vi "task.vi"() -> ()   [LabVIEW 2019]
uses:
  <vilib>/DAQmx/read.llb/DAQmx Read.vi
  <vilib>/DAQmx/read.llb/DAQmx Read (Analog 1D Wfm NChan NSamp).vi
  <vilib>/DAQmx/miscellaneous.llb/DAQmx Fill In Error Info.vi
panel:
  out "data":waveform(dbl)[](graph) caption="数据"
  in  "stop":bool caption="停止"
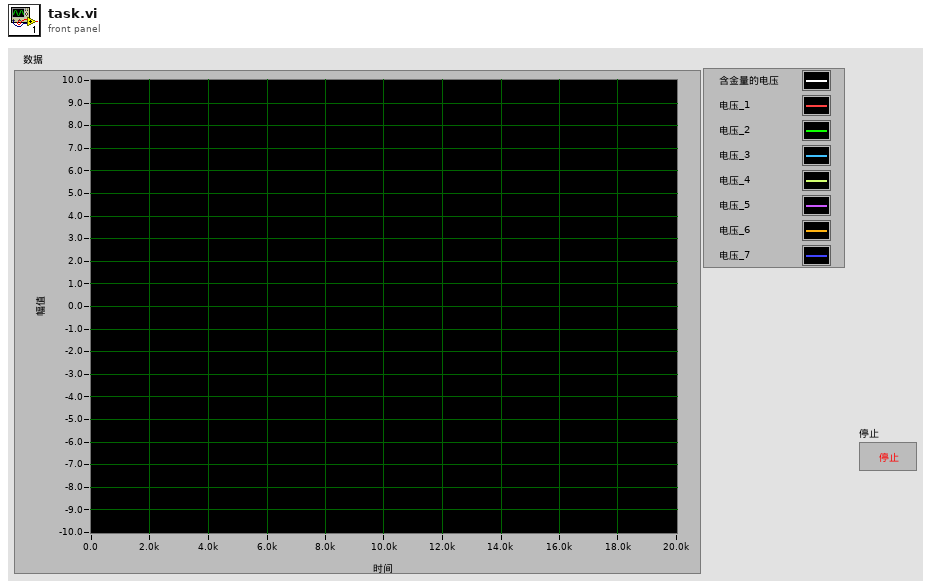
[diagram p1: front panel]
types:
  T1 = enum16{"open", "open or create", "create or replace", "create", "open (read-only)"}
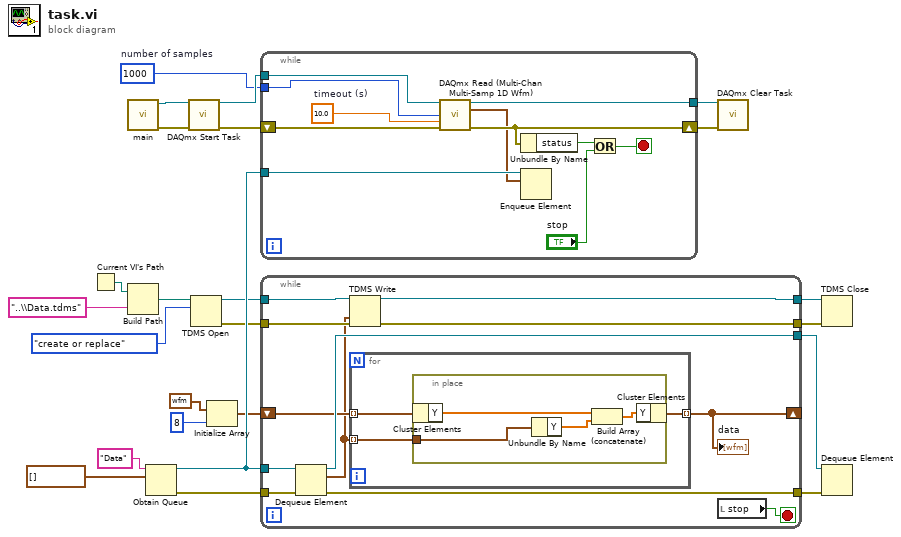
[diagram p0: block diagram]
diagram:
  w22 = 1000  # number of samples
  n1 = Current VI's Path() -> (path=w7:path)
  n2 = call "main.vi"() -> ("error out"=w18:errorcluster, "task out"=w19:refnum<k21>)  [unwired: 10 in]
  n3 = Build Path(base path=w7, name or relative path="..\\Data.tdms" ("名称或相对路径")) -> (appended path=w5:path)
  n4 = Obtain Queue(name (unnamed)="Data" ("名称（未命名）"), element data type=waveform(dbl)[] [] ("data")) -> (queue out=w14:refnum<queue>, error out=w15:errorcluster)  [unwired: 3 in, 1 out]
  n5 = call <vilib>:"DAQmx Start Task.vi"("task/channels in"=w19, "error in"=w18) -> ("task out"=w24:refnum<k21>, "error out"=w23:errorcluster)  [unwired: 12 in]
  n6 = TDMS Open(10:T1."create or replace" ("操作(0:open)"), 11:w5) -> (0:w3:errorcluster, 3:w8:refnum<k34>)  [unwired: 5 in]
  n7 = Initialize Array(waveform(dbl) {"t0"=timestamp(0 s since 1904-01-01), "dt"=0.0, "Y"=[]} ("data"), 8 ("维数大小")) -> (w9:waveform(dbl)[])
  n8 = while "While循环" {
    tunnel: w24 -> [w35]
    tunnel: w22 -> [w32]
    tunnel: [w33] -> w20
    shift-right: [w30] -> w21
    shift-left: w23 -> [w34]
    tunnel: w14 -> [w26]
    stop <- w29 stop-if-true
    w27 = 10.0  # timeout (s)
    n9 = call-poly "DAQmx Read (Multi-Chan Multi-Samp 1D Wfm).vi"("task/channels in"=w35, "number of samples per channel"=w32, "timeout"=w27, "error in"=w34) -> ("task out"=w33:refnum<k21>, "data"=w25:waveform(dbl)[], "error out"=w30:errorcluster)  [unwired: 9 in]
    n10 = Unbundle By Name(w30) -> ("status"=w31:bool)
    n11 = Enqueue Element(queue=w26, element=w25) -> ()  [unwired: 2 in, 3 out]
    n12 = Or(x=w31, y="stop") -> (x .or. y?=w29:bool)
  }
  n13 = while {
    tunnel: w15 -> [w47]
    tunnel: w14 -> [w46]
    tunnel: [w45] -> w13
    tunnel: [w44] -> w12
    shift-right: [w41] -> _
    shift-left: w9 -> [w42]
    tunnel: w8 -> [w40]
    tunnel: w3 -> [w39]
    tunnel: [w38] -> w2
    tunnel: [w37] -> w1
    stop <- w43 stop-if-true
    n14 = Dequeue Element(queue=w46, error in (no error)=w47) -> (queue out=w45:refnum<queue>, element=w36:waveform(dbl)[], error out=w44:errorcluster)  [unwired: 1 in, 1 out]
    n15 = TDMS Write(0:w40, 9:w36, 11:w39) -> (4:w37:refnum<k34>, 15:w38:errorcluster)  [unwired: 3 in, 2 out]
    n16 = for {
      tunnel: w36 -> [w48] mode=indexing
      tunnel: w42 -> [w50] mode=indexing
      tunnel: [w49] -> w41 mode=indexing
      n17 = in-place {
        in-place-border: w48 -> [w52]
        n18 = in-place-cluster #1(w50) -> ("Y"=w54:dbl[])
        n19 = Unbundle By Name(w52) -> ("Y"=w51:dbl[])
        n20 = Build Array (concatenate)(w54, w51) -> (w53:dbl[])
        n21 = in-place-cluster #1("Y"=w53) -> (w49:waveform(dbl))
      }
    }
    "data" <- w41
    n22 = local read "stop"() -> (w43:bool)
  }
  n23 = call <vilib>:"DAQmx Clear Task.vi"("task in"=w20, "error in"=w21) -> ()  [unwired: 13 in, 1 out]
  n24 = TDMS Close(8:w2, 11:w1) -> ()  [unwired: 2 out]
  n25 = Dequeue Element(queue=w13, error in (no error)=w12) -> ()  [unwired: 1 in, 4 out]
